vi "collectAI_tt.vi"() -> ()   [LabVIEW 2013]
uses:
  <vilib>/DAQmx/read.llb/DAQmx Read (Analog 2D I16 NChan NSamp).vi
  <vilib>/DAQmx/miscellaneous.llb/DAQmx Fill In Error Info.vi
panel:
  out "AIarray 2":bool[](array[boolean])
  out "AI?":bool
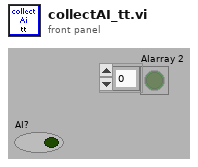
[diagram p1: front panel]
types:
  T1 = cluster{"StageS":i32, "StageL":i32, "data dir":path, "image OD":u16, "contour OD":u16, "point OD":u16, "AOlines":tag[], "AIlines":tag[], "CI lines":tag[], "DO lines":tag[], "AO names":string[], "CI names":string[], "AI names":string[], "DO names":string[]}
  T2 = typedef "LVRectTypeDef.ctl" = cluster{"Left":i16, "Top":i16, "Right":i16, "Bottom":i16}
  T3 = cluster{"Xpixels":i32, "Vxminref":dbl, "Vxmaxref":dbl, "P":dbl, "Ypixels":i32, "Vyminref":dbl, "Vymaxref":dbl, "srate":sgl, "sAOxy":i32, "timeout":dbl, "type":string, "date":string, "time":string, "Colormap":u16, "Drawing Mode":u16, "Scanning Mode":u16, "square pixels":bool, "square matrix":bool, "Xpixels Img":i32, "Vx-min Img":dbl, "VX-max Img":dbl, "Ypixels Img":i32, "Vy-min Img":dbl, "Vy-max Img ":dbl, "Angle Img":dbl, "autoshutter":bool, "finite":bool, "cont":bool, "wavdet":bool, "measpoints":i32, "avpp":i32, "bufferAO":i32, "bufferAI":i32, "starttick":u32, "waveform":path, "Vx-ref":dbl, "Vy-ref":dbl, "refreshrate":dbl, "refreshbuffer":i32, "tt_cycles":i32, "motorref":refnum<k7>, "mirrorswitch":refnum<k7>, "sample mode":i32, "maxbufferAI":i32, "sampletreshold":dbl, "srateAODO":sgl, "bin":sgl, "Pel":sgl, "Angle draw":dbl, "srate Img":sgl, "ROIimg_plotbounds":T2, "auto OD":bool, "ODfilt":u16, "reset AO_DO":bool, "aAI":i32[], "aCI":i32[], "aAO":i32[], "aDO":i32[]}
  T4 = cluster{" AI":refnum<k21>, "E_AI":errorcluster, "header":dbl[]}
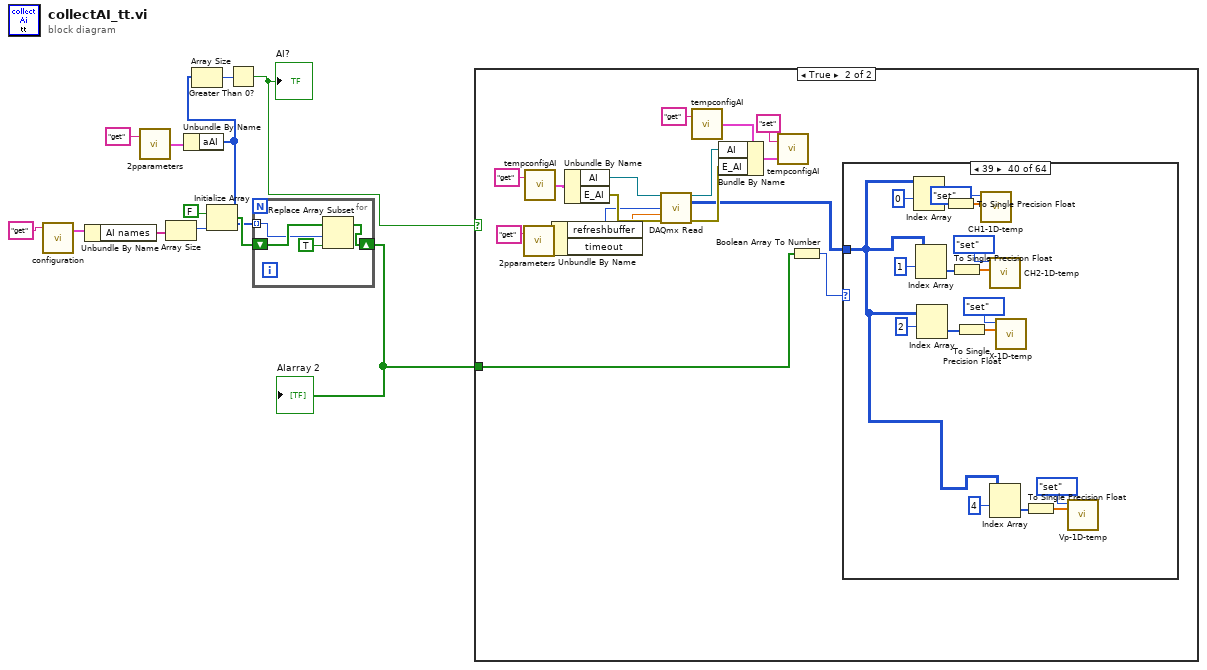
[diagram p0: block diagram]
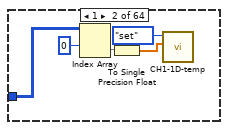
[diagram p4: hidden frame]
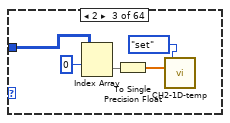
[diagram p5: hidden frame]
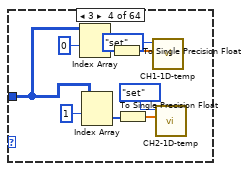
[diagram p6: hidden frame]
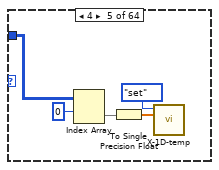
[diagram p7: hidden frame]
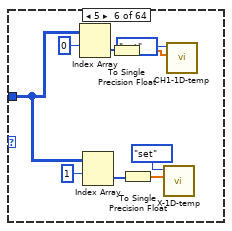
[diagram p8: hidden frame]
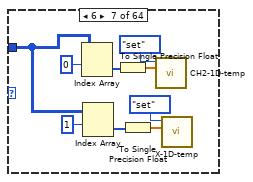
[diagram p9: hidden frame]
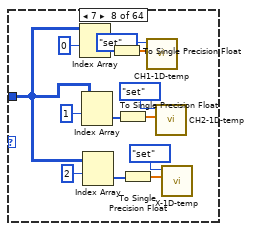
[diagram p10: hidden frame]
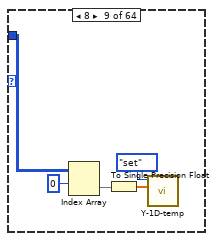
[diagram p11: hidden frame]
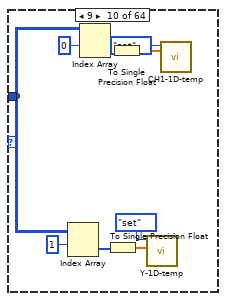
[diagram p12: hidden frame]
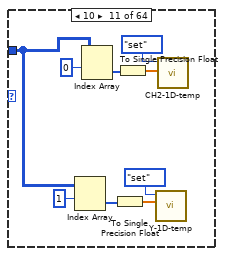
[diagram p13: hidden frame]
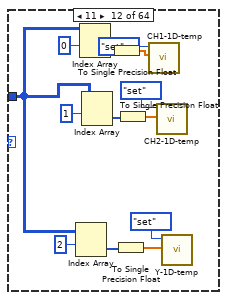
[diagram p14: hidden frame]
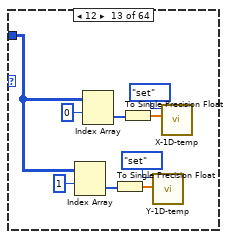
[diagram p15: hidden frame]
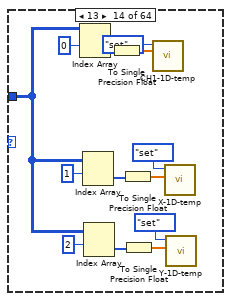
[diagram p16: hidden frame]
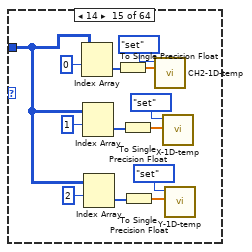
[diagram p17: hidden frame]
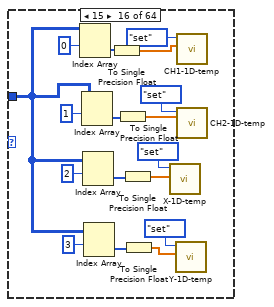
[diagram p18: hidden frame]
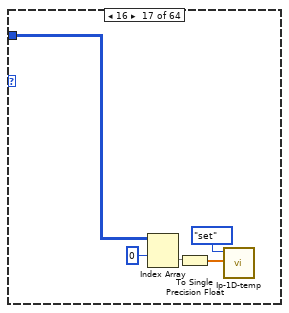
[diagram p19: hidden frame]
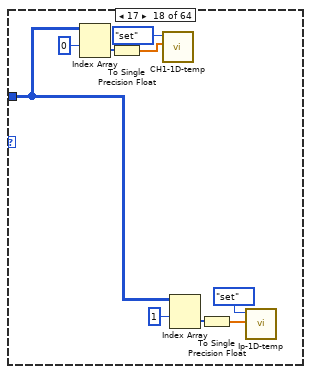
[diagram p20: hidden frame]
diagram:
  n1 = call "configuration.vi"("command"="get") -> ("config out"=w9:T1)  [unwired: 2 in, 1 out]
  n2 = Unbundle By Name(w9) -> ("AI names"=w8:string[])
  n3 = call "2pparameters.vi"("command"="get") -> ("params out"=w10:T3)  [unwired: 1 in]
  n4 = Array Size(array=w8) -> (size(s)=w7:i32)
  n5 = Unbundle By Name(w10) -> ("aAI"=w4:i32[])
  n6 = Array Size(array=w4) -> (size(s)=w3:i32)
  n7 = Initialize Array(FALSE, w7) -> (w5:bool[])
  n8 = Greater Than 0?(x=w3) -> (x > 0?=w2:bool)
  "AI?" <- w2
  n9 = for {
    tunnel: w4 -> [w15] mode=indexing
    shift-right: [w13] -> w1
    shift-left: w5 -> [w16]
    n10 = Replace Array Subset(array=w16, new element=TRUE ("new element/subarray"), index=w15) -> (w13:bool[])
  }
  "AIarray 2" <- w1
  n11 = case shown="True" w2 {
    tunnel: w1 -> [_ w18]
    frame False {
    }
    frame True {
      n12 = call "2pparameters.vi"("command"="get") -> ("params out"=w20:T3)  [unwired: 1 in]
      n13 = call "tempconfigAI.vi"("command"="get") -> ("Temp Config out"=w30:T4)  [unwired: 1 in]
      n14 = Unbundle By Name(w20) -> ("refreshbuffer"=w23:i32, "timeout"=w22:dbl)
      n15 = Unbundle By Name(w30) -> ("AI"=w29:refnum<k21>, "E_AI"=w28:errorcluster)
      n16 = call-poly <vilib>:"DAQmx Read.vi"("task/channels in"=w29, "number of samples per channel"=w23, "timeout"=w22, "error in"=w28) -> ("task out"=w24:refnum<k21>, "data"=w17:i16[][], "error out"=w33:errorcluster)  [unwired: 9 in]
      n17 = call "tempconfigAI.vi"("command"="get") -> ("Temp Config out"=w25:T4)  [unwired: 1 in]
      n18 = Bundle By Name(cluster=w25, "AI"=w24, "E_AI"=w33) -> (w32:T4)
      n19 = call "tempconfigAI.vi"("Temp Config in"=w32, "command"="set") -> ()  [unwired: 1 out]
      n20 = Boolean Array To Number(Boolean array=w18) -> (number=w19:u32)
      n21 = case shown="39" w19 {
        tunnel: w17 -> [_ w38 w43 w52 w57 w62 w71 w88 w93 w102 w111 w124 w129 w146 w159 w176 w177 w182 w191 w200 w213 w222 w235 w248 w265 w274 w287 w300 w317 w330 w347 w364 w385 w390 w399 w408 w421 w430 w443 w456 w473 w482 w495 w508 w525 w538 w555 w572 w593 w602 w615 w628 w645 w658 w675 w692 w713 w726 w743 w760 w781 w798 w819 w840]
        frame 0, Default {
        }
        frame 1 {
          n22 = Index Array(array=w38, index (row)=0) -> (element=w36:i16[])  [unwired: 1 in]
          n23 = To Single Precision Float(number=w36) -> (single precision float=w34:sgl[])
          n24 = call "CH1-1D-temp.vi"("array in"=w34, "command"=enum16{"get", "set", "clear", "append"}."set") -> ()  [unwired: 2 in, 2 out]
        }
        frame 2 {
          n25 = Index Array(array=w43, index (row)=0) -> (element=w41:i16[])  [unwired: 1 in]
          n26 = To Single Precision Float(number=w41) -> (single precision float=w40:sgl[])
          n27 = call "CH2-1D-temp.vi"("array in"=w40, "command"=enum16{"get", "set", "clear", "append"}."set") -> ()  [unwired: 2 in, 2 out]
        }
        frame 3 {
          n28 = Index Array(array=w52, index (row)=0) -> (element=w49:i16[])  [unwired: 1 in]
          n29 = Index Array(array=w52, index (row)=1) -> (element=w48:i16[])  [unwired: 1 in]
          n30 = To Single Precision Float(number=w49) -> (single precision float=w46:sgl[])
          n31 = To Single Precision Float(number=w48) -> (single precision float=w44:sgl[])
          n32 = call "CH1-1D-temp.vi"("array in"=w46, "command"=enum16{"get", "set", "clear", "append"}."set") -> ()  [unwired: 2 in, 2 out]
          n33 = call "CH2-1D-temp.vi"("array in"=w44, "command"=enum16{"get", "set", "clear", "append"}."set") -> ()  [unwired: 2 in, 2 out]
        }
        frame 4 {
          n34 = Index Array(array=w57, index (row)=0) -> (element=w55:i16[])  [unwired: 1 in]
          n35 = To Single Precision Float(number=w55) -> (single precision float=w53:sgl[])
          n36 = call "X-1D-temp.vi"("array in"=w53, "command"=enum16{"get", "set", "clear", "append"}."set") -> ()  [unwired: 2 in, 2 out]
        }
        frame 5 {
          n37 = Index Array(array=w62, index (row)=0) -> (element=w64:i16[])  [unwired: 1 in]
          n38 = Index Array(array=w62, index (row)=1) -> (element=w63:i16[])  [unwired: 1 in]
          n39 = To Single Precision Float(number=w64) -> (single precision float=w60:sgl[])
          n40 = To Single Precision Float(number=w63) -> (single precision float=w58:sgl[])
          n41 = call "X-1D-temp.vi"("array in"=w58, "command"=enum16{"get", "set", "clear", "append"}."set") -> ()  [unwired: 2 in, 2 out]
          n42 = call "CH1-1D-temp.vi"("array in"=w60, "command"=enum16{"get", "set", "clear", "append"}."set") -> ()  [unwired: 2 in, 2 out]
        }
        frame 6 {
          n43 = Index Array(array=w71, index (row)=0) -> (element=w73:i16[])  [unwired: 1 in]
          n44 = Index Array(array=w71, index (row)=1) -> (element=w72:i16[])  [unwired: 1 in]
          n45 = To Single Precision Float(number=w73) -> (single precision float=w69:sgl[])
          n46 = To Single Precision Float(number=w72) -> (single precision float=w67:sgl[])
          n47 = call "CH2-1D-temp.vi"("array in"=w69, "command"=enum16{"get", "set", "clear", "append"}."set") -> ()  [unwired: 2 in, 2 out]
          n48 = call "X-1D-temp.vi"("array in"=w67, "command"=enum16{"get", "set", "clear", "append"}."set") -> ()  [unwired: 2 in, 2 out]
        }
        frame 7 {
          n49 = Index Array(array=w88, index (row)=0) -> (element=w84:i16[])  [unwired: 1 in]
          n50 = Index Array(array=w88, index (row)=1) -> (element=w83:i16[])  [unwired: 1 in]
          n51 = Index Array(array=w88, index (row)=2) -> (element=w82:i16[])  [unwired: 1 in]
          n52 = To Single Precision Float(number=w84) -> (single precision float=w80:sgl[])
          n53 = To Single Precision Float(number=w83) -> (single precision float=w78:sgl[])
          n54 = To Single Precision Float(number=w82) -> (single precision float=w76:sgl[])
          n55 = call "CH1-1D-temp.vi"("array in"=w80, "command"=enum16{"get", "set", "clear", "append"}."set") -> ()  [unwired: 2 in, 2 out]
          n56 = call "CH2-1D-temp.vi"("array in"=w78, "command"=enum16{"get", "set", "clear", "append"}."set") -> ()  [unwired: 2 in, 2 out]
          n57 = call "X-1D-temp.vi"("array in"=w76, "command"=enum16{"get", "set", "clear", "append"}."set") -> ()  [unwired: 2 in, 2 out]
        }
        frame 8 {
          n58 = Index Array(array=w93, index (row)=0) -> (element=w92:i16[])  [unwired: 1 in]
          n59 = To Single Precision Float(number=w92) -> (single precision float=w89:sgl[])
          n60 = call "Y-1D-temp.vi"("array in"=w89, "command"=enum16{"get", "set", "clear", "append"}."set") -> ()  [unwired: 2 in, 2 out]
        }
        frame 9 {
          n61 = Index Array(array=w102, index (row)=1) -> (element=w99:i16[])  [unwired: 1 in]
          n62 = Index Array(array=w102, index (row)=0) -> (element=w100:i16[])  [unwired: 1 in]
          n63 = To Single Precision Float(number=w99) -> (single precision float=w94:sgl[])
          n64 = To Single Precision Float(number=w100) -> (single precision float=w96:sgl[])
          n65 = call "Y-1D-temp.vi"("array in"=w94, "command"=enum16{"get", "set", "clear", "append"}."set") -> ()  [unwired: 2 in, 2 out]
          n66 = call "CH1-1D-temp.vi"("array in"=w96, "command"=enum16{"get", "set", "clear", "append"}."set") -> ()  [unwired: 2 in, 2 out]
        }
        frame 10 {
          n67 = Index Array(array=w111, index (row)=1) -> (element=w108:i16[])  [unwired: 1 in]
          n68 = Index Array(array=w111, index (row)=0) -> (element=w109:i16[])  [unwired: 1 in]
          n69 = To Single Precision Float(number=w108) -> (single precision float=w103:sgl[])
          n70 = To Single Precision Float(number=w109) -> (single precision float=w106:sgl[])
          n71 = call "Y-1D-temp.vi"("array in"=w103, "command"=enum16{"get", "set", "clear", "append"}."set") -> ()  [unwired: 2 in, 2 out]
          n72 = call "CH2-1D-temp.vi"("array in"=w106, "command"=enum16{"get", "set", "clear", "append"}."set") -> ()  [unwired: 2 in, 2 out]
        }
        frame 11 {
          n73 = Index Array(array=w124, index (row)=2) -> (element=w119:i16[])  [unwired: 1 in]
          n74 = Index Array(array=w124, index (row)=0) -> (element=w121:i16[])  [unwired: 1 in]
          n75 = Index Array(array=w124, index (row)=1) -> (element=w120:i16[])  [unwired: 1 in]
          n76 = To Single Precision Float(number=w121) -> (single precision float=w116:sgl[])
          n77 = To Single Precision Float(number=w119) -> (single precision float=w113:sgl[])
          n78 = To Single Precision Float(number=w120) -> (single precision float=w114:sgl[])
          n79 = call "CH1-1D-temp.vi"("array in"=w116, "command"=enum16{"get", "set", "clear", "append"}."set") -> ()  [unwired: 2 in, 2 out]
          n80 = call "CH2-1D-temp.vi"("array in"=w114, "command"=enum16{"get", "set", "clear", "append"}."set") -> ()  [unwired: 2 in, 2 out]
          n81 = call "Y-1D-temp.vi"("array in"=w113, "command"=enum16{"get", "set", "clear", "append"}."set") -> ()  [unwired: 2 in, 2 out]
        }
        frame 12 {
          n82 = Index Array(array=w129, index (row)=1) -> (element=w131:i16[])  [unwired: 1 in]
          n83 = Index Array(array=w129, index (row)=0) -> (element=w132:i16[])  [unwired: 1 in]
          n84 = To Single Precision Float(number=w131) -> (single precision float=w125:sgl[])
          n85 = To Single Precision Float(number=w132) -> (single precision float=w127:sgl[])
          n86 = call "Y-1D-temp.vi"("array in"=w125, "command"=enum16{"get", "set", "clear", "append"}."set") -> ()  [unwired: 2 in, 2 out]
          n87 = call "X-1D-temp.vi"("array in"=w127, "command"=enum16{"get", "set", "clear", "append"}."set") -> ()  [unwired: 2 in, 2 out]
        }
        frame 13 {
          n88 = Index Array(array=w146, index (row)=0) -> (element=w143:i16[])  [unwired: 1 in]
          n89 = Index Array(array=w146, index (row)=1) -> (element=w142:i16[])  [unwired: 1 in]
          n90 = Index Array(array=w146, index (row)=2) -> (element=w141:i16[])  [unwired: 1 in]
          n91 = To Single Precision Float(number=w143) -> (single precision float=w138:sgl[])
          n92 = To Single Precision Float(number=w142) -> (single precision float=w136:sgl[])
          n93 = To Single Precision Float(number=w141) -> (single precision float=w134:sgl[])
          n94 = call "CH1-1D-temp.vi"("array in"=w138, "command"=enum16{"get", "set", "clear", "append"}."set") -> ()  [unwired: 2 in, 2 out]
          n95 = call "X-1D-temp.vi"("array in"=w136, "command"=enum16{"get", "set", "clear", "append"}."set") -> ()  [unwired: 2 in, 2 out]
          n96 = call "Y-1D-temp.vi"("array in"=w134, "command"=enum16{"get", "set", "clear", "append"}."set") -> ()  [unwired: 2 in, 2 out]
        }
        frame 14 {
          n97 = Index Array(array=w159, index (row)=0) -> (element=w156:i16[])  [unwired: 1 in]
          n98 = Index Array(array=w159, index (row)=1) -> (element=w155:i16[])  [unwired: 1 in]
          n99 = Index Array(array=w159, index (row)=2) -> (element=w154:i16[])  [unwired: 1 in]
          n100 = To Single Precision Float(number=w156) -> (single precision float=w151:sgl[])
          n101 = To Single Precision Float(number=w155) -> (single precision float=w149:sgl[])
          n102 = To Single Precision Float(number=w154) -> (single precision float=w147:sgl[])
          n103 = call "CH2-1D-temp.vi"("array in"=w151, "command"=enum16{"get", "set", "clear", "append"}."set") -> ()  [unwired: 2 in, 2 out]
          n104 = call "X-1D-temp.vi"("array in"=w149, "command"=enum16{"get", "set", "clear", "append"}."set") -> ()  [unwired: 2 in, 2 out]
          n105 = call "Y-1D-temp.vi"("array in"=w147, "command"=enum16{"get", "set", "clear", "append"}."set") -> ()  [unwired: 2 in, 2 out]
        }
        frame 15 {
          n106 = Index Array(array=w176, index (row)=0) -> (element=w172:i16[])  [unwired: 1 in]
          n107 = Index Array(array=w176, index (row)=1) -> (element=w171:i16[])  [unwired: 1 in]
          n108 = Index Array(array=w176, index (row)=2) -> (element=w170:i16[])  [unwired: 1 in]
          n109 = Index Array(array=w176, index (row)=3) -> (element=w169:i16[])  [unwired: 1 in]
          n110 = To Single Precision Float(number=w172) -> (single precision float=w166:sgl[])
          n111 = To Single Precision Float(number=w171) -> (single precision float=w164:sgl[])
          n112 = To Single Precision Float(number=w170) -> (single precision float=w162:sgl[])
          n113 = To Single Precision Float(number=w169) -> (single precision float=w160:sgl[])
          n114 = call "X-1D-temp.vi"("array in"=w162, "command"=enum16{"get", "set", "clear", "append"}."set") -> ()  [unwired: 2 in, 2 out]
          n115 = call "Y-1D-temp.vi"("array in"=w160, "command"=enum16{"get", "set", "clear", "append"}."set") -> ()  [unwired: 2 in, 2 out]
          n116 = call "CH1-1D-temp.vi"("array in"=w166, "command"=enum16{"get", "set", "clear", "append"}."set") -> ()  [unwired: 2 in, 2 out]
          n117 = call "CH2-1D-temp.vi"("array in"=w164, "command"=enum16{"get", "set", "clear", "append"}."set") -> ()  [unwired: 2 in, 2 out]
        }
        frame 16 {
          n118 = Index Array(array=w177, index (row)=0) -> (element=w180:i16[])  [unwired: 1 in]
          n119 = To Single Precision Float(number=w180) -> (single precision float=w178:sgl[])
          n120 = call "Ip-1D-temp.vi"("array in"=w178, "command"=enum16{"get", "set", "clear", "append"}."set") -> ()  [unwired: 2 in, 2 out]
        }
        frame 17 {
          n121 = Index Array(array=w182, index (row)=0) -> (element=w189:i16[])  [unwired: 1 in]
          n122 = To Single Precision Float(number=w189) -> (single precision float=w187:sgl[])
          n123 = call "CH1-1D-temp.vi"("array in"=w187, "command"=enum16{"get", "set", "clear", "append"}."set") -> ()  [unwired: 2 in, 2 out]
          n124 = Index Array(array=w182, index (row)=1) -> (element=w185:i16[])  [unwired: 1 in]
          n125 = To Single Precision Float(number=w185) -> (single precision float=w183:sgl[])
          n126 = call "Ip-1D-temp.vi"("array in"=w183, "command"=enum16{"get", "set", "clear", "append"}."set") -> ()  [unwired: 2 in, 2 out]
        }
        frame 18 {
          n127 = Index Array(array=w191, index (row)=0) -> (element=w198:i16[])  [unwired: 1 in]
          n128 = To Single Precision Float(number=w198) -> (single precision float=w197:sgl[])
          n129 = Index Array(array=w191, index (row)=1) -> (element=w194:i16[])  [unwired: 1 in]
          n130 = call "CH2-1D-temp.vi"("array in"=w197, "command"=enum16{"get", "set", "clear", "append"}."set") -> ()  [unwired: 2 in, 2 out]
          n131 = To Single Precision Float(number=w194) -> (single precision float=w192:sgl[])
          n132 = call "Ip-1D-temp.vi"("array in"=w192, "command"=enum16{"get", "set", "clear", "append"}."set") -> ()  [unwired: 2 in, 2 out]
        }
        frame 19 {
          n133 = Index Array(array=w200, index (row)=0) -> (element=w210:i16[])  [unwired: 1 in]
          n134 = Index Array(array=w200, index (row)=1) -> (element=w209:i16[])  [unwired: 1 in]
          n135 = To Single Precision Float(number=w210) -> (single precision float=w207:sgl[])
          n136 = To Single Precision Float(number=w209) -> (single precision float=w205:sgl[])
          n137 = call "CH1-1D-temp.vi"("array in"=w207, "command"=enum16{"get", "set", "clear", "append"}."set") -> ()  [unwired: 2 in, 2 out]
          n138 = call "CH2-1D-temp.vi"("array in"=w205, "command"=enum16{"get", "set", "clear", "append"}."set") -> ()  [unwired: 2 in, 2 out]
          n139 = Index Array(array=w200, index (row)=2) -> (element=w203:i16[])  [unwired: 1 in]
          n140 = To Single Precision Float(number=w203) -> (single precision float=w201:sgl[])
          n141 = call "Ip-1D-temp.vi"("array in"=w201, "command"=enum16{"get", "set", "clear", "append"}."set") -> ()  [unwired: 2 in, 2 out]
        }
        frame 20 {
          n142 = Index Array(array=w213, index (row)=0) -> (element=w220:i16[])  [unwired: 1 in]
          n143 = To Single Precision Float(number=w220) -> (single precision float=w218:sgl[])
          n144 = Index Array(array=w213, index (row)=1) -> (element=w216:i16[])  [unwired: 1 in]
          n145 = call "X-1D-temp.vi"("array in"=w218, "command"=enum16{"get", "set", "clear", "append"}."set") -> ()  [unwired: 2 in, 2 out]
          n146 = To Single Precision Float(number=w216) -> (single precision float=w214:sgl[])
          n147 = call "Ip-1D-temp.vi"("array in"=w214, "command"=enum16{"get", "set", "clear", "append"}."set") -> ()  [unwired: 2 in, 2 out]
        }
        frame 21 {
          n148 = Index Array(array=w222, index (row)=0) -> (element=w232:i16[])  [unwired: 1 in]
          n149 = Index Array(array=w222, index (row)=1) -> (element=w231:i16[])  [unwired: 1 in]
          n150 = To Single Precision Float(number=w232) -> (single precision float=w229:sgl[])
          n151 = To Single Precision Float(number=w231) -> (single precision float=w227:sgl[])
          n152 = Index Array(array=w222, index (row)=2) -> (element=w225:i16[])  [unwired: 1 in]
          n153 = call "X-1D-temp.vi"("array in"=w227, "command"=enum16{"get", "set", "clear", "append"}."set") -> ()  [unwired: 2 in, 2 out]
          n154 = call "CH1-1D-temp.vi"("array in"=w229, "command"=enum16{"get", "set", "clear", "append"}."set") -> ()  [unwired: 2 in, 2 out]
          n155 = To Single Precision Float(number=w225) -> (single precision float=w223:sgl[])
          n156 = call "Ip-1D-temp.vi"("array in"=w223, "command"=enum16{"get", "set", "clear", "append"}."set") -> ()  [unwired: 2 in, 2 out]
        }
        frame 22 {
          n157 = Index Array(array=w235, index (row)=0) -> (element=w245:i16[])  [unwired: 1 in]
          n158 = Index Array(array=w235, index (row)=1) -> (element=w244:i16[])  [unwired: 1 in]
          n159 = To Single Precision Float(number=w245) -> (single precision float=w242:sgl[])
          n160 = To Single Precision Float(number=w244) -> (single precision float=w240:sgl[])
          n161 = Index Array(array=w235, index (row)=2) -> (element=w238:i16[])  [unwired: 1 in]
          n162 = call "CH2-1D-temp.vi"("array in"=w242, "command"=enum16{"get", "set", "clear", "append"}."set") -> ()  [unwired: 2 in, 2 out]
          n163 = To Single Precision Float(number=w238) -> (single precision float=w236:sgl[])
          n164 = call "X-1D-temp.vi"("array in"=w240, "command"=enum16{"get", "set", "clear", "append"}."set") -> ()  [unwired: 2 in, 2 out]
          n165 = call "Ip-1D-temp.vi"("array in"=w236, "command"=enum16{"get", "set", "clear", "append"}."set") -> ()  [unwired: 2 in, 2 out]
        }
        frame 23 {
          n166 = Index Array(array=w248, index (row)=0) -> (element=w261:i16[])  [unwired: 1 in]
          n167 = Index Array(array=w248, index (row)=1) -> (element=w260:i16[])  [unwired: 1 in]
          n168 = Index Array(array=w248, index (row)=2) -> (element=w259:i16[])  [unwired: 1 in]
          n169 = To Single Precision Float(number=w261) -> (single precision float=w257:sgl[])
          n170 = To Single Precision Float(number=w260) -> (single precision float=w255:sgl[])
          n171 = To Single Precision Float(number=w259) -> (single precision float=w253:sgl[])
          n172 = call "CH1-1D-temp.vi"("array in"=w257, "command"=enum16{"get", "set", "clear", "append"}."set") -> ()  [unwired: 2 in, 2 out]
          n173 = Index Array(array=w248, index (row)=3) -> (element=w251:i16[])  [unwired: 1 in]
          n174 = call "CH2-1D-temp.vi"("array in"=w255, "command"=enum16{"get", "set", "clear", "append"}."set") -> ()  [unwired: 2 in, 2 out]
          n175 = call "X-1D-temp.vi"("array in"=w253, "command"=enum16{"get", "set", "clear", "append"}."set") -> ()  [unwired: 2 in, 2 out]
          n176 = To Single Precision Float(number=w251) -> (single precision float=w249:sgl[])
          n177 = call "Ip-1D-temp.vi"("array in"=w249, "command"=enum16{"get", "set", "clear", "append"}."set") -> ()  [unwired: 2 in, 2 out]
        }
        frame 24 {
          n178 = Index Array(array=w265, index (row)=0) -> (element=w273:i16[])  [unwired: 1 in]
          n179 = To Single Precision Float(number=w273) -> (single precision float=w270:sgl[])
          n180 = call "Y-1D-temp.vi"("array in"=w270, "command"=enum16{"get", "set", "clear", "append"}."set") -> ()  [unwired: 2 in, 2 out]
          n181 = Index Array(array=w265, index (row)=1) -> (element=w268:i16[])  [unwired: 1 in]
          n182 = To Single Precision Float(number=w268) -> (single precision float=w266:sgl[])
          n183 = call "Ip-1D-temp.vi"("array in"=w266, "command"=enum16{"get", "set", "clear", "append"}."set") -> ()  [unwired: 2 in, 2 out]
        }
        frame 25 {
          n184 = Index Array(array=w274, index (row)=1) -> (element=w284:i16[])  [unwired: 1 in]
          n185 = Index Array(array=w274, index (row)=0) -> (element=w285:i16[])  [unwired: 1 in]
          n186 = To Single Precision Float(number=w284) -> (single precision float=w279:sgl[])
          n187 = To Single Precision Float(number=w285) -> (single precision float=w281:sgl[])
          n188 = call "Y-1D-temp.vi"("array in"=w279, "command"=enum16{"get", "set", "clear", "append"}."set") -> ()  [unwired: 2 in, 2 out]
          n189 = call "CH1-1D-temp.vi"("array in"=w281, "command"=enum16{"get", "set", "clear", "append"}."set") -> ()  [unwired: 2 in, 2 out]
          n190 = Index Array(array=w274, index (row)=2) -> (element=w277:i16[])  [unwired: 1 in]
          n191 = To Single Precision Float(number=w277) -> (single precision float=w275:sgl[])
          n192 = call "Ip-1D-temp.vi"("array in"=w275, "command"=enum16{"get", "set", "clear", "append"}."set") -> ()  [unwired: 2 in, 2 out]
        }
        frame 26 {
          n193 = Index Array(array=w287, index (row)=1) -> (element=w297:i16[])  [unwired: 1 in]
          n194 = Index Array(array=w287, index (row)=0) -> (element=w298:i16[])  [unwired: 1 in]
          n195 = To Single Precision Float(number=w297) -> (single precision float=w292:sgl[])
          n196 = To Single Precision Float(number=w298) -> (single precision float=w295:sgl[])
          n197 = call "Y-1D-temp.vi"("array in"=w292, "command"=enum16{"get", "set", "clear", "append"}."set") -> ()  [unwired: 2 in, 2 out]
          n198 = call "CH2-1D-temp.vi"("array in"=w295, "command"=enum16{"get", "set", "clear", "append"}."set") -> ()  [unwired: 2 in, 2 out]
          n199 = Index Array(array=w287, index (row)=2) -> (element=w290:i16[])  [unwired: 1 in]
          n200 = To Single Precision Float(number=w290) -> (single precision float=w288:sgl[])
          n201 = call "Ip-1D-temp.vi"("array in"=w288, "command"=enum16{"get", "set", "clear", "append"}."set") -> ()  [unwired: 2 in, 2 out]
        }
        frame 27 {
          n202 = Index Array(array=w300, index (row)=2) -> (element=w312:i16[])  [unwired: 1 in]
          n203 = Index Array(array=w300, index (row)=0) -> (element=w314:i16[])  [unwired: 1 in]
          n204 = Index Array(array=w300, index (row)=1) -> (element=w313:i16[])  [unwired: 1 in]
          n205 = To Single Precision Float(number=w314) -> (single precision float=w309:sgl[])
          n206 = To Single Precision Float(number=w312) -> (single precision float=w306:sgl[])
          n207 = To Single Precision Float(number=w313) -> (single precision float=w307:sgl[])
          n208 = call "CH1-1D-temp.vi"("array in"=w309, "command"=enum16{"get", "set", "clear", "append"}."set") -> ()  [unwired: 2 in, 2 out]
          n209 = call "CH2-1D-temp.vi"("array in"=w307, "command"=enum16{"get", "set", "clear", "append"}."set") -> ()  [unwired: 2 in, 2 out]
          n210 = Index Array(array=w300, index (row)=3) -> (element=w303:i16[])  [unwired: 1 in]
          n211 = call "Y-1D-temp.vi"("array in"=w306, "command"=enum16{"get", "set", "clear", "append"}."set") -> ()  [unwired: 2 in, 2 out]
          n212 = To Single Precision Float(number=w303) -> (single precision float=w301:sgl[])
          n213 = call "Ip-1D-temp.vi"("array in"=w301, "command"=enum16{"get", "set", "clear", "append"}."set") -> ()  [unwired: 2 in, 2 out]
        }
        frame 28 {
          n214 = Index Array(array=w317, index (row)=1) -> (element=w327:i16[])  [unwired: 1 in]
          n215 = Index Array(array=w317, index (row)=0) -> (element=w328:i16[])  [unwired: 1 in]
          n216 = To Single Precision Float(number=w327) -> (single precision float=w322:sgl[])
          n217 = To Single Precision Float(number=w328) -> (single precision float=w324:sgl[])
          n218 = call "Y-1D-temp.vi"("array in"=w322, "command"=enum16{"get", "set", "clear", "append"}."set") -> ()  [unwired: 2 in, 2 out]
          n219 = Index Array(array=w317, index (row)=2) -> (element=w320:i16[])  [unwired: 1 in]
          n220 = call "X-1D-temp.vi"("array in"=w324, "command"=enum16{"get", "set", "clear", "append"}."set") -> ()  [unwired: 2 in, 2 out]
          n221 = To Single Precision Float(number=w320) -> (single precision float=w318:sgl[])
          n222 = call "Ip-1D-temp.vi"("array in"=w318, "command"=enum16{"get", "set", "clear", "append"}."set") -> ()  [unwired: 2 in, 2 out]
        }
        frame 29 {
          n223 = Index Array(array=w330, index (row)=0) -> (element=w344:i16[])  [unwired: 1 in]
          n224 = Index Array(array=w330, index (row)=1) -> (element=w343:i16[])  [unwired: 1 in]
          n225 = Index Array(array=w330, index (row)=2) -> (element=w342:i16[])  [unwired: 1 in]
          n226 = To Single Precision Float(number=w344) -> (single precision float=w339:sgl[])
          n227 = To Single Precision Float(number=w343) -> (single precision float=w337:sgl[])
          n228 = To Single Precision Float(number=w342) -> (single precision float=w335:sgl[])
          n229 = Index Array(array=w330, index (row)=3) -> (element=w333:i16[])  [unwired: 1 in]
          n230 = call "CH1-1D-temp.vi"("array in"=w339, "command"=enum16{"get", "set", "clear", "append"}."set") -> ()  [unwired: 2 in, 2 out]
          n231 = call "X-1D-temp.vi"("array in"=w337, "command"=enum16{"get", "set", "clear", "append"}."set") -> ()  [unwired: 2 in, 2 out]
          n232 = call "Y-1D-temp.vi"("array in"=w335, "command"=enum16{"get", "set", "clear", "append"}."set") -> ()  [unwired: 2 in, 2 out]
          n233 = To Single Precision Float(number=w333) -> (single precision float=w331:sgl[])
          n234 = call "Ip-1D-temp.vi"("array in"=w331, "command"=enum16{"get", "set", "clear", "append"}."set") -> ()  [unwired: 2 in, 2 out]
        }
        frame 30 {
          n235 = Index Array(array=w347, index (row)=3) -> (element=w350:i16[])  [unwired: 1 in]
          n236 = Index Array(array=w347, index (row)=0) -> (element=w361:i16[])  [unwired: 1 in]
          n237 = Index Array(array=w347, index (row)=1) -> (element=w360:i16[])  [unwired: 1 in]
          n238 = Index Array(array=w347, index (row)=2) -> (element=w359:i16[])  [unwired: 1 in]
          n239 = To Single Precision Float(number=w350) -> (single precision float=w348:sgl[])
          n240 = To Single Precision Float(number=w361) -> (single precision float=w356:sgl[])
          n241 = To Single Precision Float(number=w360) -> (single precision float=w354:sgl[])
          n242 = To Single Precision Float(number=w359) -> (single precision float=w352:sgl[])
          n243 = call "CH2-1D-temp.vi"("array in"=w356, "command"=enum16{"get", "set", "clear", "append"}."set") -> ()  [unwired: 2 in, 2 out]
          n244 = call "Ip-1D-temp.vi"("array in"=w348, "command"=enum16{"get", "set", "clear", "append"}."set") -> ()  [unwired: 2 in, 2 out]
          n245 = call "X-1D-temp.vi"("array in"=w354, "command"=enum16{"get", "set", "clear", "append"}."set") -> ()  [unwired: 2 in, 2 out]
          n246 = call "Y-1D-temp.vi"("array in"=w352, "command"=enum16{"get", "set", "clear", "append"}."set") -> ()  [unwired: 2 in, 2 out]
        }
        frame 31 {
          n247 = Index Array(array=w364, index (row)=0) -> (element=w381:i16[])  [unwired: 1 in]
          n248 = Index Array(array=w364, index (row)=1) -> (element=w380:i16[])  [unwired: 1 in]
          n249 = Index Array(array=w364, index (row)=2) -> (element=w379:i16[])  [unwired: 1 in]
          n250 = Index Array(array=w364, index (row)=3) -> (element=w378:i16[])  [unwired: 1 in]
          n251 = Index Array(array=w364, index (row)=4) -> (element=w367:i16[])  [unwired: 1 in]
          n252 = To Single Precision Float(number=w381) -> (single precision float=w375:sgl[])
          n253 = To Single Precision Float(number=w380) -> (single precision float=w373:sgl[])
          n254 = To Single Precision Float(number=w367) -> (single precision float=w365:sgl[])
          n255 = To Single Precision Float(number=w379) -> (single precision float=w371:sgl[])
          n256 = To Single Precision Float(number=w378) -> (single precision float=w369:sgl[])
          n257 = call "Ip-1D-temp.vi"("array in"=w365, "command"=enum16{"get", "set", "clear", "append"}."set") -> ()  [unwired: 2 in, 2 out]
          n258 = call "X-1D-temp.vi"("array in"=w371, "command"=enum16{"get", "set", "clear", "append"}."set") -> ()  [unwired: 2 in, 2 out]
          n259 = call "Y-1D-temp.vi"("array in"=w369, "command"=enum16{"get", "set", "clear", "append"}."set") -> ()  [unwired: 2 in, 2 out]
          n260 = call "CH1-1D-temp.vi"("array in"=w375, "command"=enum16{"get", "set", "clear", "append"}."set") -> ()  [unwired: 2 in, 2 out]
          n261 = call "CH2-1D-temp.vi"("array in"=w373, "command"=enum16{"get", "set", "clear", "append"}."set") -> ()  [unwired: 2 in, 2 out]
        }
        frame 32 {
          n262 = Index Array(array=w385, index (row)=1) -> (element=w388:i16[])  [unwired: 1 in]
          n263 = To Single Precision Float(number=w388) -> (single precision float=w386:sgl[])
          n264 = call "Vp-1D-temp.vi"("array in"=w386, "command"=enum16{"get", "set", "clear", "append"}."set") -> ()  [unwired: 2 in, 2 out]
        }
        frame 33 {
          n265 = Index Array(array=w390, index (row)=0) -> (element=w397:i16[])  [unwired: 1 in]
          n266 = To Single Precision Float(number=w397) -> (single precision float=w395:sgl[])
          n267 = call "CH1-1D-temp.vi"("array in"=w395, "command"=enum16{"get", "set", "clear", "append"}."set") -> ()  [unwired: 2 in, 2 out]
          n268 = Index Array(array=w390, index (row)=2) -> (element=w393:i16[])  [unwired: 1 in]
          n269 = To Single Precision Float(number=w393) -> (single precision float=w391:sgl[])
          n270 = call "Vp-1D-temp.vi"("array in"=w391, "command"=enum16{"get", "set", "clear", "append"}."set") -> ()  [unwired: 2 in, 2 out]
        }
        frame 34 {
          n271 = Index Array(array=w399, index (row)=0) -> (element=w406:i16[])  [unwired: 1 in]
          n272 = To Single Precision Float(number=w406) -> (single precision float=w405:sgl[])
          n273 = Index Array(array=w399, index (row)=2) -> (element=w402:i16[])  [unwired: 1 in]
          n274 = call "CH2-1D-temp.vi"("array in"=w405, "command"=enum16{"get", "set", "clear", "append"}."set") -> ()  [unwired: 2 in, 2 out]
          n275 = To Single Precision Float(number=w402) -> (single precision float=w400:sgl[])
          n276 = call "Vp-1D-temp.vi"("array in"=w400, "command"=enum16{"get", "set", "clear", "append"}."set") -> ()  [unwired: 2 in, 2 out]
        }
        frame 35 {
          n277 = Index Array(array=w408, index (row)=0) -> (element=w418:i16[])  [unwired: 1 in]
          n278 = Index Array(array=w408, index (row)=1) -> (element=w417:i16[])  [unwired: 1 in]
          n279 = To Single Precision Float(number=w418) -> (single precision float=w415:sgl[])
          n280 = To Single Precision Float(number=w417) -> (single precision float=w413:sgl[])
          n281 = call "CH1-1D-temp.vi"("array in"=w415, "command"=enum16{"get", "set", "clear", "append"}."set") -> ()  [unwired: 2 in, 2 out]
          n282 = call "CH2-1D-temp.vi"("array in"=w413, "command"=enum16{"get", "set", "clear", "append"}."set") -> ()  [unwired: 2 in, 2 out]
          n283 = Index Array(array=w408, index (row)=3) -> (element=w411:i16[])  [unwired: 1 in]
          n284 = To Single Precision Float(number=w411) -> (single precision float=w409:sgl[])
          n285 = call "Vp-1D-temp.vi"("array in"=w409, "command"=enum16{"get", "set", "clear", "append"}."set") -> ()  [unwired: 2 in, 2 out]
        }
        frame 36 {
          n286 = Index Array(array=w421, index (row)=0) -> (element=w428:i16[])  [unwired: 1 in]
          n287 = To Single Precision Float(number=w428) -> (single precision float=w426:sgl[])
          n288 = Index Array(array=w421, index (row)=2) -> (element=w424:i16[])  [unwired: 1 in]
          n289 = call "X-1D-temp.vi"("array in"=w426, "command"=enum16{"get", "set", "clear", "append"}."set") -> ()  [unwired: 2 in, 2 out]
          n290 = To Single Precision Float(number=w424) -> (single precision float=w422:sgl[])
          n291 = call "Vp-1D-temp.vi"("array in"=w422, "command"=enum16{"get", "set", "clear", "append"}."set") -> ()  [unwired: 2 in, 2 out]
        }
        frame 37 {
          n292 = Index Array(array=w430, index (row)=0) -> (element=w440:i16[])  [unwired: 1 in]
          n293 = Index Array(array=w430, index (row)=1) -> (element=w439:i16[])  [unwired: 1 in]
          n294 = To Single Precision Float(number=w440) -> (single precision float=w437:sgl[])
          n295 = To Single Precision Float(number=w439) -> (single precision float=w435:sgl[])
          n296 = Index Array(array=w430, index (row)=3) -> (element=w433:i16[])  [unwired: 1 in]
          n297 = call "X-1D-temp.vi"("array in"=w435, "command"=enum16{"get", "set", "clear", "append"}."set") -> ()  [unwired: 2 in, 2 out]
          n298 = call "CH1-1D-temp.vi"("array in"=w437, "command"=enum16{"get", "set", "clear", "append"}."set") -> ()  [unwired: 2 in, 2 out]
          n299 = To Single Precision Float(number=w433) -> (single precision float=w431:sgl[])
          n300 = call "Vp-1D-temp.vi"("array in"=w431, "command"=enum16{"get", "set", "clear", "append"}."set") -> ()  [unwired: 2 in, 2 out]
        }
        frame 38 {
          n301 = Index Array(array=w443, index (row)=0) -> (element=w453:i16[])  [unwired: 1 in]
          n302 = Index Array(array=w443, index (row)=1) -> (element=w452:i16[])  [unwired: 1 in]
          n303 = To Single Precision Float(number=w453) -> (single precision float=w450:sgl[])
          n304 = To Single Precision Float(number=w452) -> (single precision float=w448:sgl[])
          n305 = Index Array(array=w443, index (row)=3) -> (element=w446:i16[])  [unwired: 1 in]
          n306 = call "CH2-1D-temp.vi"("array in"=w450, "command"=enum16{"get", "set", "clear", "append"}."set") -> ()  [unwired: 2 in, 2 out]
          n307 = call "X-1D-temp.vi"("array in"=w448, "command"=enum16{"get", "set", "clear", "append"}."set") -> ()  [unwired: 2 in, 2 out]
          n308 = To Single Precision Float(number=w446) -> (single precision float=w444:sgl[])
          n309 = call "Vp-1D-temp.vi"("array in"=w444, "command"=enum16{"get", "set", "clear", "append"}."set") -> ()  [unwired: 2 in, 2 out]
        }
        frame 39 {
          n310 = Index Array(array=w456, index (row)=0) -> (element=w469:i16[])  [unwired: 1 in]
          n311 = Index Array(array=w456, index (row)=1) -> (element=w468:i16[])  [unwired: 1 in]
          n312 = Index Array(array=w456, index (row)=2) -> (element=w467:i16[])  [unwired: 1 in]
          n313 = To Single Precision Float(number=w469) -> (single precision float=w465:sgl[])
          n314 = To Single Precision Float(number=w468) -> (single precision float=w463:sgl[])
          n315 = To Single Precision Float(number=w467) -> (single precision float=w461:sgl[])
          n316 = call "CH1-1D-temp.vi"("array in"=w465, "command"=enum16{"get", "set", "clear", "append"}."set") -> ()  [unwired: 2 in, 2 out]
          n317 = call "CH2-1D-temp.vi"("array in"=w463, "command"=enum16{"get", "set", "clear", "append"}."set") -> ()  [unwired: 2 in, 2 out]
          n318 = Index Array(array=w456, index (row)=4) -> (element=w459:i16[])  [unwired: 1 in]
          n319 = call "X-1D-temp.vi"("array in"=w461, "command"=enum16{"get", "set", "clear", "append"}."set") -> ()  [unwired: 2 in, 2 out]
          n320 = To Single Precision Float(number=w459) -> (single precision float=w457:sgl[])
          n321 = call "Vp-1D-temp.vi"("array in"=w457, "command"=enum16{"get", "set", "clear", "append"}."set") -> ()  [unwired: 2 in, 2 out]
        }
        frame 40 {
          n322 = Index Array(array=w473, index (row)=0) -> (element=w481:i16[])  [unwired: 1 in]
          n323 = To Single Precision Float(number=w481) -> (single precision float=w478:sgl[])
          n324 = call "Y-1D-temp.vi"("array in"=w478, "command"=enum16{"get", "set", "clear", "append"}."set") -> ()  [unwired: 2 in, 2 out]
          n325 = Index Array(array=w473, index (row)=2) -> (element=w476:i16[])  [unwired: 1 in]
          n326 = To Single Precision Float(number=w476) -> (single precision float=w474:sgl[])
          n327 = call "Vp-1D-temp.vi"("array in"=w474, "command"=enum16{"get", "set", "clear", "append"}."set") -> ()  [unwired: 2 in, 2 out]
        }
        frame 41 {
          n328 = Index Array(array=w482, index (row)=1) -> (element=w492:i16[])  [unwired: 1 in]
          n329 = Index Array(array=w482, index (row)=0) -> (element=w493:i16[])  [unwired: 1 in]
          n330 = To Single Precision Float(number=w492) -> (single precision float=w487:sgl[])
          n331 = To Single Precision Float(number=w493) -> (single precision float=w489:sgl[])
          n332 = call "Y-1D-temp.vi"("array in"=w487, "command"=enum16{"get", "set", "clear", "append"}."set") -> ()  [unwired: 2 in, 2 out]
          n333 = call "CH1-1D-temp.vi"("array in"=w489, "command"=enum16{"get", "set", "clear", "append"}."set") -> ()  [unwired: 2 in, 2 out]
          n334 = Index Array(array=w482, index (row)=3) -> (element=w485:i16[])  [unwired: 1 in]
          n335 = To Single Precision Float(number=w485) -> (single precision float=w483:sgl[])
          n336 = call "Vp-1D-temp.vi"("array in"=w483, "command"=enum16{"get", "set", "clear", "append"}."set") -> ()  [unwired: 2 in, 2 out]
        }
        frame 42 {
          n337 = Index Array(array=w495, index (row)=1) -> (element=w505:i16[])  [unwired: 1 in]
          n338 = Index Array(array=w495, index (row)=0) -> (element=w506:i16[])  [unwired: 1 in]
          n339 = To Single Precision Float(number=w505) -> (single precision float=w500:sgl[])
          n340 = To Single Precision Float(number=w506) -> (single precision float=w503:sgl[])
          n341 = call "Y-1D-temp.vi"("array in"=w500, "command"=enum16{"get", "set", "clear", "append"}."set") -> ()  [unwired: 2 in, 2 out]
          n342 = call "CH2-1D-temp.vi"("array in"=w503, "command"=enum16{"get", "set", "clear", "append"}."set") -> ()  [unwired: 2 in, 2 out]
          n343 = Index Array(array=w495, index (row)=3) -> (element=w498:i16[])  [unwired: 1 in]
          n344 = To Single Precision Float(number=w498) -> (single precision float=w496:sgl[])
          n345 = call "Vp-1D-temp.vi"("array in"=w496, "command"=enum16{"get", "set", "clear", "append"}."set") -> ()  [unwired: 2 in, 2 out]
        }
        frame 43 {
          n346 = Index Array(array=w508, index (row)=2) -> (element=w520:i16[])  [unwired: 1 in]
          n347 = Index Array(array=w508, index (row)=0) -> (element=w522:i16[])  [unwired: 1 in]
          n348 = Index Array(array=w508, index (row)=1) -> (element=w521:i16[])  [unwired: 1 in]
          n349 = To Single Precision Float(number=w522) -> (single precision float=w517:sgl[])
          n350 = To Single Precision Float(number=w520) -> (single precision float=w514:sgl[])
          n351 = To Single Precision Float(number=w521) -> (single precision float=w515:sgl[])
          n352 = call "CH1-1D-temp.vi"("array in"=w517, "command"=enum16{"get", "set", "clear", "append"}."set") -> ()  [unwired: 2 in, 2 out]
          n353 = call "CH2-1D-temp.vi"("array in"=w515, "command"=enum16{"get", "set", "clear", "append"}."set") -> ()  [unwired: 2 in, 2 out]
          n354 = call "Y-1D-temp.vi"("array in"=w514, "command"=enum16{"get", "set", "clear", "append"}."set") -> ()  [unwired: 2 in, 2 out]
          n355 = Index Array(array=w508, index (row)=4) -> (element=w511:i16[])  [unwired: 1 in]
          n356 = To Single Precision Float(number=w511) -> (single precision float=w509:sgl[])
          n357 = call "Vp-1D-temp.vi"("array in"=w509, "command"=enum16{"get", "set", "clear", "append"}."set") -> ()  [unwired: 2 in, 2 out]
        }
        frame 44 {
          n358 = Index Array(array=w525, index (row)=1) -> (element=w535:i16[])  [unwired: 1 in]
          n359 = Index Array(array=w525, index (row)=0) -> (element=w536:i16[])  [unwired: 1 in]
          n360 = To Single Precision Float(number=w535) -> (single precision float=w530:sgl[])
          n361 = To Single Precision Float(number=w536) -> (single precision float=w532:sgl[])
          n362 = call "Y-1D-temp.vi"("array in"=w530, "command"=enum16{"get", "set", "clear", "append"}."set") -> ()  [unwired: 2 in, 2 out]
          n363 = Index Array(array=w525, index (row)=3) -> (element=w528:i16[])  [unwired: 1 in]
          n364 = call "X-1D-temp.vi"("array in"=w532, "command"=enum16{"get", "set", "clear", "append"}."set") -> ()  [unwired: 2 in, 2 out]
          n365 = To Single Precision Float(number=w528) -> (single precision float=w526:sgl[])
          n366 = call "Vp-1D-temp.vi"("array in"=w526, "command"=enum16{"get", "set", "clear", "append"}."set") -> ()  [unwired: 2 in, 2 out]
        }
        frame 45 {
          n367 = Index Array(array=w538, index (row)=0) -> (element=w552:i16[])  [unwired: 1 in]
          n368 = Index Array(array=w538, index (row)=1) -> (element=w551:i16[])  [unwired: 1 in]
          n369 = Index Array(array=w538, index (row)=2) -> (element=w550:i16[])  [unwired: 1 in]
          n370 = To Single Precision Float(number=w552) -> (single precision float=w547:sgl[])
          n371 = To Single Precision Float(number=w551) -> (single precision float=w545:sgl[])
          n372 = To Single Precision Float(number=w550) -> (single precision float=w543:sgl[])
          n373 = Index Array(array=w538, index (row)=4) -> (element=w541:i16[])  [unwired: 1 in]
          n374 = call "CH1-1D-temp.vi"("array in"=w547, "command"=enum16{"get", "set", "clear", "append"}."set") -> ()  [unwired: 2 in, 2 out]
          n375 = call "X-1D-temp.vi"("array in"=w545, "command"=enum16{"get", "set", "clear", "append"}."set") -> ()  [unwired: 2 in, 2 out]
          n376 = call "Y-1D-temp.vi"("array in"=w543, "command"=enum16{"get", "set", "clear", "append"}."set") -> ()  [unwired: 2 in, 2 out]
          n377 = To Single Precision Float(number=w541) -> (single precision float=w539:sgl[])
          n378 = call "Vp-1D-temp.vi"("array in"=w539, "command"=enum16{"get", "set", "clear", "append"}."set") -> ()  [unwired: 2 in, 2 out]
        }
        frame 46 {
          n379 = Index Array(array=w555, index (row)=0) -> (element=w569:i16[])  [unwired: 1 in]
          n380 = Index Array(array=w555, index (row)=1) -> (element=w568:i16[])  [unwired: 1 in]
          n381 = Index Array(array=w555, index (row)=4) -> (element=w558:i16[])  [unwired: 1 in]
          n382 = Index Array(array=w555, index (row)=2) -> (element=w567:i16[])  [unwired: 1 in]
          n383 = To Single Precision Float(number=w569) -> (single precision float=w564:sgl[])
          n384 = To Single Precision Float(number=w558) -> (single precision float=w556:sgl[])
          n385 = To Single Precision Float(number=w568) -> (single precision float=w562:sgl[])
          n386 = To Single Precision Float(number=w567) -> (single precision float=w560:sgl[])
          n387 = call "CH2-1D-temp.vi"("array in"=w564, "command"=enum16{"get", "set", "clear", "append"}."set") -> ()  [unwired: 2 in, 2 out]
          n388 = call "Vp-1D-temp.vi"("array in"=w556, "command"=enum16{"get", "set", "clear", "append"}."set") -> ()  [unwired: 2 in, 2 out]
          n389 = call "X-1D-temp.vi"("array in"=w562, "command"=enum16{"get", "set", "clear", "append"}."set") -> ()  [unwired: 2 in, 2 out]
          n390 = call "Y-1D-temp.vi"("array in"=w560, "command"=enum16{"get", "set", "clear", "append"}."set") -> ()  [unwired: 2 in, 2 out]
        }
        frame 47 {
          n391 = Index Array(array=w572, index (row)=0) -> (element=w589:i16[])  [unwired: 1 in]
          n392 = Index Array(array=w572, index (row)=1) -> (element=w588:i16[])  [unwired: 1 in]
          n393 = Index Array(array=w572, index (row)=2) -> (element=w587:i16[])  [unwired: 1 in]
          n394 = Index Array(array=w572, index (row)=3) -> (element=w586:i16[])  [unwired: 1 in]
          n395 = Index Array(array=w572, index (row)=5) -> (element=w575:i16[])  [unwired: 1 in]
          n396 = To Single Precision Float(number=w589) -> (single precision float=w583:sgl[])
          n397 = To Single Precision Float(number=w588) -> (single precision float=w581:sgl[])
          n398 = To Single Precision Float(number=w587) -> (single precision float=w579:sgl[])
          n399 = To Single Precision Float(number=w586) -> (single precision float=w577:sgl[])
          n400 = To Single Precision Float(number=w575) -> (single precision float=w573:sgl[])
          n401 = call "Vp-1D-temp.vi"("array in"=w573, "command"=enum16{"get", "set", "clear", "append"}."set") -> ()  [unwired: 2 in, 2 out]
          n402 = call "X-1D-temp.vi"("array in"=w579, "command"=enum16{"get", "set", "clear", "append"}."set") -> ()  [unwired: 2 in, 2 out]
          n403 = call "Y-1D-temp.vi"("array in"=w577, "command"=enum16{"get", "set", "clear", "append"}."set") -> ()  [unwired: 2 in, 2 out]
          n404 = call "CH1-1D-temp.vi"("array in"=w583, "command"=enum16{"get", "set", "clear", "append"}."set") -> ()  [unwired: 2 in, 2 out]
          n405 = call "CH2-1D-temp.vi"("array in"=w581, "command"=enum16{"get", "set", "clear", "append"}."set") -> ()  [unwired: 2 in, 2 out]
        }
        frame 48 {
          n406 = Index Array(array=w593, index (row)=0) -> (element=w599:i16[])  [unwired: 1 in]
          n407 = Index Array(array=w593, index (row)=1) -> (element=w598:i16[])  [unwired: 1 in]
          n408 = To Single Precision Float(number=w599) -> (single precision float=w596:sgl[])
          n409 = To Single Precision Float(number=w598) -> (single precision float=w594:sgl[])
          n410 = call "Ip-1D-temp.vi"("array in"=w596, "command"=enum16{"get", "set", "clear", "append"}."set") -> ()  [unwired: 2 in, 2 out]
          n411 = call "Vp-1D-temp.vi"("array in"=w594, "command"=enum16{"get", "set", "clear", "append"}."set") -> ()  [unwired: 2 in, 2 out]
        }
        frame 49 {
          n412 = Index Array(array=w602, index (row)=0) -> (element=w613:i16[])  [unwired: 1 in]
          n413 = To Single Precision Float(number=w613) -> (single precision float=w611:sgl[])
          n414 = call "CH1-1D-temp.vi"("array in"=w611, "command"=enum16{"get", "set", "clear", "append"}."set") -> ()  [unwired: 2 in, 2 out]
          n415 = Index Array(array=w602, index (row)=1) -> (element=w608:i16[])  [unwired: 1 in]
          n416 = Index Array(array=w602, index (row)=2) -> (element=w607:i16[])  [unwired: 1 in]
          n417 = To Single Precision Float(number=w608) -> (single precision float=w605:sgl[])
          n418 = To Single Precision Float(number=w607) -> (single precision float=w603:sgl[])
          n419 = call "Ip-1D-temp.vi"("array in"=w605, "command"=enum16{"get", "set", "clear", "append"}."set") -> ()  [unwired: 2 in, 2 out]
          n420 = call "Vp-1D-temp.vi"("array in"=w603, "command"=enum16{"get", "set", "clear", "append"}."set") -> ()  [unwired: 2 in, 2 out]
        }
        frame 50 {
          n421 = Index Array(array=w615, index (row)=0) -> (element=w626:i16[])  [unwired: 1 in]
          n422 = To Single Precision Float(number=w626) -> (single precision float=w625:sgl[])
          n423 = Index Array(array=w615, index (row)=1) -> (element=w621:i16[])  [unwired: 1 in]
          n424 = Index Array(array=w615, index (row)=2) -> (element=w620:i16[])  [unwired: 1 in]
          n425 = call "CH2-1D-temp.vi"("array in"=w625, "command"=enum16{"get", "set", "clear", "append"}."set") -> ()  [unwired: 2 in, 2 out]
          n426 = To Single Precision Float(number=w621) -> (single precision float=w618:sgl[])
          n427 = To Single Precision Float(number=w620) -> (single precision float=w616:sgl[])
          n428 = call "Ip-1D-temp.vi"("array in"=w618, "command"=enum16{"get", "set", "clear", "append"}."set") -> ()  [unwired: 2 in, 2 out]
          n429 = call "Vp-1D-temp.vi"("array in"=w616, "command"=enum16{"get", "set", "clear", "append"}."set") -> ()  [unwired: 2 in, 2 out]
        }
        frame 51 {
          n430 = Index Array(array=w628, index (row)=0) -> (element=w642:i16[])  [unwired: 1 in]
          n431 = Index Array(array=w628, index (row)=1) -> (element=w641:i16[])  [unwired: 1 in]
          n432 = To Single Precision Float(number=w642) -> (single precision float=w639:sgl[])
          n433 = To Single Precision Float(number=w641) -> (single precision float=w637:sgl[])
          n434 = call "CH1-1D-temp.vi"("array in"=w639, "command"=enum16{"get", "set", "clear", "append"}."set") -> ()  [unwired: 2 in, 2 out]
          n435 = call "CH2-1D-temp.vi"("array in"=w637, "command"=enum16{"get", "set", "clear", "append"}."set") -> ()  [unwired: 2 in, 2 out]
          n436 = Index Array(array=w628, index (row)=2) -> (element=w634:i16[])  [unwired: 1 in]
          n437 = Index Array(array=w628, index (row)=3) -> (element=w633:i16[])  [unwired: 1 in]
          n438 = To Single Precision Float(number=w634) -> (single precision float=w631:sgl[])
          n439 = To Single Precision Float(number=w633) -> (single precision float=w629:sgl[])
          n440 = call "Ip-1D-temp.vi"("array in"=w631, "command"=enum16{"get", "set", "clear", "append"}."set") -> ()  [unwired: 2 in, 2 out]
          n441 = call "Vp-1D-temp.vi"("array in"=w629, "command"=enum16{"get", "set", "clear", "append"}."set") -> ()  [unwired: 2 in, 2 out]
        }
        frame 52 {
          n442 = Index Array(array=w645, index (row)=0) -> (element=w656:i16[])  [unwired: 1 in]
          n443 = To Single Precision Float(number=w656) -> (single precision float=w654:sgl[])
          n444 = Index Array(array=w645, index (row)=1) -> (element=w651:i16[])  [unwired: 1 in]
          n445 = Index Array(array=w645, index (row)=2) -> (element=w650:i16[])  [unwired: 1 in]
          n446 = call "X-1D-temp.vi"("array in"=w654, "command"=enum16{"get", "set", "clear", "append"}."set") -> ()  [unwired: 2 in, 2 out]
          n447 = To Single Precision Float(number=w651) -> (single precision float=w648:sgl[])
          n448 = To Single Precision Float(number=w650) -> (single precision float=w646:sgl[])
          n449 = call "Ip-1D-temp.vi"("array in"=w648, "command"=enum16{"get", "set", "clear", "append"}."set") -> ()  [unwired: 2 in, 2 out]
          n450 = call "Vp-1D-temp.vi"("array in"=w646, "command"=enum16{"get", "set", "clear", "append"}."set") -> ()  [unwired: 2 in, 2 out]
        }
        frame 53 {
          n451 = Index Array(array=w658, index (row)=0) -> (element=w672:i16[])  [unwired: 1 in]
          n452 = Index Array(array=w658, index (row)=1) -> (element=w671:i16[])  [unwired: 1 in]
          n453 = To Single Precision Float(number=w672) -> (single precision float=w669:sgl[])
          n454 = To Single Precision Float(number=w671) -> (single precision float=w667:sgl[])
          n455 = Index Array(array=w658, index (row)=2) -> (element=w664:i16[])  [unwired: 1 in]
          n456 = Index Array(array=w658, index (row)=3) -> (element=w663:i16[])  [unwired: 1 in]
          n457 = call "X-1D-temp.vi"("array in"=w667, "command"=enum16{"get", "set", "clear", "append"}."set") -> ()  [unwired: 2 in, 2 out]
          n458 = call "CH1-1D-temp.vi"("array in"=w669, "command"=enum16{"get", "set", "clear", "append"}."set") -> ()  [unwired: 2 in, 2 out]
          n459 = To Single Precision Float(number=w664) -> (single precision float=w661:sgl[])
          n460 = To Single Precision Float(number=w663) -> (single precision float=w659:sgl[])
          n461 = call "Ip-1D-temp.vi"("array in"=w661, "command"=enum16{"get", "set", "clear", "append"}."set") -> ()  [unwired: 2 in, 2 out]
          n462 = call "Vp-1D-temp.vi"("array in"=w659, "command"=enum16{"get", "set", "clear", "append"}."set") -> ()  [unwired: 2 in, 2 out]
        }
        frame 54 {
          n463 = Index Array(array=w675, index (row)=0) -> (element=w689:i16[])  [unwired: 1 in]
          n464 = Index Array(array=w675, index (row)=1) -> (element=w688:i16[])  [unwired: 1 in]
          n465 = To Single Precision Float(number=w689) -> (single precision float=w686:sgl[])
          n466 = To Single Precision Float(number=w688) -> (single precision float=w684:sgl[])
          n467 = Index Array(array=w675, index (row)=2) -> (element=w681:i16[])  [unwired: 1 in]
          n468 = Index Array(array=w675, index (row)=3) -> (element=w680:i16[])  [unwired: 1 in]
          n469 = call "CH2-1D-temp.vi"("array in"=w686, "command"=enum16{"get", "set", "clear", "append"}."set") -> ()  [unwired: 2 in, 2 out]
          n470 = To Single Precision Float(number=w681) -> (single precision float=w678:sgl[])
          n471 = call "X-1D-temp.vi"("array in"=w684, "command"=enum16{"get", "set", "clear", "append"}."set") -> ()  [unwired: 2 in, 2 out]
          n472 = To Single Precision Float(number=w680) -> (single precision float=w676:sgl[])
          n473 = call "Ip-1D-temp.vi"("array in"=w678, "command"=enum16{"get", "set", "clear", "append"}."set") -> ()  [unwired: 2 in, 2 out]
          n474 = call "Vp-1D-temp.vi"("array in"=w676, "command"=enum16{"get", "set", "clear", "append"}."set") -> ()  [unwired: 2 in, 2 out]
        }
        frame 55 {
          n475 = Index Array(array=w692, index (row)=0) -> (element=w709:i16[])  [unwired: 1 in]
          n476 = Index Array(array=w692, index (row)=1) -> (element=w708:i16[])  [unwired: 1 in]
          n477 = Index Array(array=w692, index (row)=2) -> (element=w707:i16[])  [unwired: 1 in]
          n478 = To Single Precision Float(number=w709) -> (single precision float=w705:sgl[])
          n479 = To Single Precision Float(number=w708) -> (single precision float=w703:sgl[])
          n480 = To Single Precision Float(number=w707) -> (single precision float=w701:sgl[])
          n481 = call "CH1-1D-temp.vi"("array in"=w705, "command"=enum16{"get", "set", "clear", "append"}."set") -> ()  [unwired: 2 in, 2 out]
          n482 = Index Array(array=w692, index (row)=3) -> (element=w698:i16[])  [unwired: 1 in]
          n483 = call "CH2-1D-temp.vi"("array in"=w703, "command"=enum16{"get", "set", "clear", "append"}."set") -> ()  [unwired: 2 in, 2 out]
          n484 = Index Array(array=w692, index (row)=4) -> (element=w697:i16[])  [unwired: 1 in]
          n485 = call "X-1D-temp.vi"("array in"=w701, "command"=enum16{"get", "set", "clear", "append"}."set") -> ()  [unwired: 2 in, 2 out]
          n486 = To Single Precision Float(number=w698) -> (single precision float=w695:sgl[])
          n487 = To Single Precision Float(number=w697) -> (single precision float=w693:sgl[])
          n488 = call "Ip-1D-temp.vi"("array in"=w695, "command"=enum16{"get", "set", "clear", "append"}."set") -> ()  [unwired: 2 in, 2 out]
          n489 = call "Vp-1D-temp.vi"("array in"=w693, "command"=enum16{"get", "set", "clear", "append"}."set") -> ()  [unwired: 2 in, 2 out]
        }
        frame 56 {
          n490 = Index Array(array=w713, index (row)=0) -> (element=w725:i16[])  [unwired: 1 in]
          n491 = To Single Precision Float(number=w725) -> (single precision float=w722:sgl[])
          n492 = call "Y-1D-temp.vi"("array in"=w722, "command"=enum16{"get", "set", "clear", "append"}."set") -> ()  [unwired: 2 in, 2 out]
          n493 = Index Array(array=w713, index (row)=1) -> (element=w719:i16[])  [unwired: 1 in]
          n494 = Index Array(array=w713, index (row)=2) -> (element=w718:i16[])  [unwired: 1 in]
          n495 = To Single Precision Float(number=w719) -> (single precision float=w716:sgl[])
          n496 = To Single Precision Float(number=w718) -> (single precision float=w714:sgl[])
          n497 = call "Ip-1D-temp.vi"("array in"=w716, "command"=enum16{"get", "set", "clear", "append"}."set") -> ()  [unwired: 2 in, 2 out]
          n498 = call "Vp-1D-temp.vi"("array in"=w714, "command"=enum16{"get", "set", "clear", "append"}."set") -> ()  [unwired: 2 in, 2 out]
        }
        frame 57 {
          n499 = Index Array(array=w726, index (row)=1) -> (element=w740:i16[])  [unwired: 1 in]
          n500 = Index Array(array=w726, index (row)=0) -> (element=w741:i16[])  [unwired: 1 in]
          n501 = To Single Precision Float(number=w740) -> (single precision float=w735:sgl[])
          n502 = To Single Precision Float(number=w741) -> (single precision float=w737:sgl[])
          n503 = call "Y-1D-temp.vi"("array in"=w735, "command"=enum16{"get", "set", "clear", "append"}."set") -> ()  [unwired: 2 in, 2 out]
          n504 = call "CH1-1D-temp.vi"("array in"=w737, "command"=enum16{"get", "set", "clear", "append"}."set") -> ()  [unwired: 2 in, 2 out]
          n505 = Index Array(array=w726, index (row)=2) -> (element=w732:i16[])  [unwired: 1 in]
          n506 = Index Array(array=w726, index (row)=3) -> (element=w731:i16[])  [unwired: 1 in]
          n507 = To Single Precision Float(number=w732) -> (single precision float=w729:sgl[])
          n508 = To Single Precision Float(number=w731) -> (single precision float=w727:sgl[])
          n509 = call "Ip-1D-temp.vi"("array in"=w729, "command"=enum16{"get", "set", "clear", "append"}."set") -> ()  [unwired: 2 in, 2 out]
          n510 = call "Vp-1D-temp.vi"("array in"=w727, "command"=enum16{"get", "set", "clear", "append"}."set") -> ()  [unwired: 2 in, 2 out]
        }
        frame 58 {
          n511 = Index Array(array=w743, index (row)=1) -> (element=w757:i16[])  [unwired: 1 in]
          n512 = Index Array(array=w743, index (row)=0) -> (element=w758:i16[])  [unwired: 1 in]
          n513 = To Single Precision Float(number=w757) -> (single precision float=w752:sgl[])
          n514 = To Single Precision Float(number=w758) -> (single precision float=w755:sgl[])
          n515 = call "Y-1D-temp.vi"("array in"=w752, "command"=enum16{"get", "set", "clear", "append"}."set") -> ()  [unwired: 2 in, 2 out]
          n516 = call "CH2-1D-temp.vi"("array in"=w755, "command"=enum16{"get", "set", "clear", "append"}."set") -> ()  [unwired: 2 in, 2 out]
          n517 = Index Array(array=w743, index (row)=2) -> (element=w749:i16[])  [unwired: 1 in]
          n518 = Index Array(array=w743, index (row)=3) -> (element=w748:i16[])  [unwired: 1 in]
          n519 = To Single Precision Float(number=w749) -> (single precision float=w746:sgl[])
          n520 = To Single Precision Float(number=w748) -> (single precision float=w744:sgl[])
          n521 = call "Ip-1D-temp.vi"("array in"=w746, "command"=enum16{"get", "set", "clear", "append"}."set") -> ()  [unwired: 2 in, 2 out]
          n522 = call "Vp-1D-temp.vi"("array in"=w744, "command"=enum16{"get", "set", "clear", "append"}."set") -> ()  [unwired: 2 in, 2 out]
        }
        frame 59 {
          n523 = Index Array(array=w760, index (row)=2) -> (element=w776:i16[])  [unwired: 1 in]
          n524 = Index Array(array=w760, index (row)=0) -> (element=w778:i16[])  [unwired: 1 in]
          n525 = Index Array(array=w760, index (row)=1) -> (element=w777:i16[])  [unwired: 1 in]
          n526 = To Single Precision Float(number=w778) -> (single precision float=w773:sgl[])
          n527 = To Single Precision Float(number=w776) -> (single precision float=w770:sgl[])
          n528 = To Single Precision Float(number=w777) -> (single precision float=w771:sgl[])
          n529 = call "CH1-1D-temp.vi"("array in"=w773, "command"=enum16{"get", "set", "clear", "append"}."set") -> ()  [unwired: 2 in, 2 out]
          n530 = call "CH2-1D-temp.vi"("array in"=w771, "command"=enum16{"get", "set", "clear", "append"}."set") -> ()  [unwired: 2 in, 2 out]
          n531 = Index Array(array=w760, index (row)=3) -> (element=w766:i16[])  [unwired: 1 in]
          n532 = call "Y-1D-temp.vi"("array in"=w770, "command"=enum16{"get", "set", "clear", "append"}."set") -> ()  [unwired: 2 in, 2 out]
          n533 = Index Array(array=w760, index (row)=4) -> (element=w765:i16[])  [unwired: 1 in]
          n534 = To Single Precision Float(number=w766) -> (single precision float=w763:sgl[])
          n535 = To Single Precision Float(number=w765) -> (single precision float=w761:sgl[])
          n536 = call "Ip-1D-temp.vi"("array in"=w763, "command"=enum16{"get", "set", "clear", "append"}."set") -> ()  [unwired: 2 in, 2 out]
          n537 = call "Vp-1D-temp.vi"("array in"=w761, "command"=enum16{"get", "set", "clear", "append"}."set") -> ()  [unwired: 2 in, 2 out]
        }
        frame 60 {
          n538 = Index Array(array=w781, index (row)=1) -> (element=w795:i16[])  [unwired: 1 in]
          n539 = Index Array(array=w781, index (row)=0) -> (element=w796:i16[])  [unwired: 1 in]
          n540 = To Single Precision Float(number=w795) -> (single precision float=w790:sgl[])
          n541 = To Single Precision Float(number=w796) -> (single precision float=w792:sgl[])
          n542 = call "Y-1D-temp.vi"("array in"=w790, "command"=enum16{"get", "set", "clear", "append"}."set") -> ()  [unwired: 2 in, 2 out]
          n543 = Index Array(array=w781, index (row)=2) -> (element=w787:i16[])  [unwired: 1 in]
          n544 = Index Array(array=w781, index (row)=3) -> (element=w786:i16[])  [unwired: 1 in]
          n545 = call "X-1D-temp.vi"("array in"=w792, "command"=enum16{"get", "set", "clear", "append"}."set") -> ()  [unwired: 2 in, 2 out]
          n546 = To Single Precision Float(number=w787) -> (single precision float=w784:sgl[])
          n547 = To Single Precision Float(number=w786) -> (single precision float=w782:sgl[])
          n548 = call "Ip-1D-temp.vi"("array in"=w784, "command"=enum16{"get", "set", "clear", "append"}."set") -> ()  [unwired: 2 in, 2 out]
          n549 = call "Vp-1D-temp.vi"("array in"=w782, "command"=enum16{"get", "set", "clear", "append"}."set") -> ()  [unwired: 2 in, 2 out]
        }
        frame 61 {
          n550 = Index Array(array=w798, index (row)=0) -> (element=w816:i16[])  [unwired: 1 in]
          n551 = Index Array(array=w798, index (row)=1) -> (element=w815:i16[])  [unwired: 1 in]
          n552 = Index Array(array=w798, index (row)=2) -> (element=w814:i16[])  [unwired: 1 in]
          n553 = To Single Precision Float(number=w816) -> (single precision float=w811:sgl[])
          n554 = To Single Precision Float(number=w815) -> (single precision float=w809:sgl[])
          n555 = To Single Precision Float(number=w814) -> (single precision float=w807:sgl[])
          n556 = Index Array(array=w798, index (row)=3) -> (element=w804:i16[])  [unwired: 1 in]
          n557 = Index Array(array=w798, index (row)=4) -> (element=w803:i16[])  [unwired: 1 in]
          n558 = call "CH1-1D-temp.vi"("array in"=w811, "command"=enum16{"get", "set", "clear", "append"}."set") -> ()  [unwired: 2 in, 2 out]
          n559 = call "X-1D-temp.vi"("array in"=w809, "command"=enum16{"get", "set", "clear", "append"}."set") -> ()  [unwired: 2 in, 2 out]
          n560 = call "Y-1D-temp.vi"("array in"=w807, "command"=enum16{"get", "set", "clear", "append"}."set") -> ()  [unwired: 2 in, 2 out]
          n561 = To Single Precision Float(number=w804) -> (single precision float=w801:sgl[])
          n562 = To Single Precision Float(number=w803) -> (single precision float=w799:sgl[])
          n563 = call "Ip-1D-temp.vi"("array in"=w801, "command"=enum16{"get", "set", "clear", "append"}."set") -> ()  [unwired: 2 in, 2 out]
          n564 = call "Vp-1D-temp.vi"("array in"=w799, "command"=enum16{"get", "set", "clear", "append"}."set") -> ()  [unwired: 2 in, 2 out]
        }
        frame 62 {
          n565 = Index Array(array=w819, index (row)=3) -> (element=w825:i16[])  [unwired: 1 in]
          n566 = Index Array(array=w819, index (row)=0) -> (element=w837:i16[])  [unwired: 1 in]
          n567 = Index Array(array=w819, index (row)=1) -> (element=w836:i16[])  [unwired: 1 in]
          n568 = Index Array(array=w819, index (row)=4) -> (element=w824:i16[])  [unwired: 1 in]
          n569 = Index Array(array=w819, index (row)=2) -> (element=w835:i16[])  [unwired: 1 in]
          n570 = To Single Precision Float(number=w825) -> (single precision float=w822:sgl[])
          n571 = To Single Precision Float(number=w837) -> (single precision float=w832:sgl[])
          n572 = To Single Precision Float(number=w824) -> (single precision float=w820:sgl[])
          n573 = To Single Precision Float(number=w836) -> (single precision float=w830:sgl[])
          n574 = To Single Precision Float(number=w835) -> (single precision float=w828:sgl[])
          n575 = call "CH2-1D-temp.vi"("array in"=w832, "command"=enum16{"get", "set", "clear", "append"}."set") -> ()  [unwired: 2 in, 2 out]
          n576 = call "Ip-1D-temp.vi"("array in"=w822, "command"=enum16{"get", "set", "clear", "append"}."set") -> ()  [unwired: 2 in, 2 out]
          n577 = call "Vp-1D-temp.vi"("array in"=w820, "command"=enum16{"get", "set", "clear", "append"}."set") -> ()  [unwired: 2 in, 2 out]
          n578 = call "X-1D-temp.vi"("array in"=w830, "command"=enum16{"get", "set", "clear", "append"}."set") -> ()  [unwired: 2 in, 2 out]
          n579 = call "Y-1D-temp.vi"("array in"=w828, "command"=enum16{"get", "set", "clear", "append"}."set") -> ()  [unwired: 2 in, 2 out]
        }
        frame 63 {
          n580 = Index Array(array=w840, index (row)=0) -> (element=w861:i16[])  [unwired: 1 in]
          n581 = Index Array(array=w840, index (row)=1) -> (element=w860:i16[])  [unwired: 1 in]
          n582 = Index Array(array=w840, index (row)=2) -> (element=w859:i16[])  [unwired: 1 in]
          n583 = Index Array(array=w840, index (row)=3) -> (element=w858:i16[])  [unwired: 1 in]
          n584 = Index Array(array=w840, index (row)=4) -> (element=w846:i16[])  [unwired: 1 in]
          n585 = Index Array(array=w840, index (row)=5) -> (element=w845:i16[])  [unwired: 1 in]
          n586 = To Single Precision Float(number=w861) -> (single precision float=w855:sgl[])
          n587 = To Single Precision Float(number=w860) -> (single precision float=w853:sgl[])
          n588 = To Single Precision Float(number=w846) -> (single precision float=w843:sgl[])
          n589 = To Single Precision Float(number=w859) -> (single precision float=w851:sgl[])
          n590 = To Single Precision Float(number=w858) -> (single precision float=w849:sgl[])
          n591 = To Single Precision Float(number=w845) -> (single precision float=w841:sgl[])
          n592 = call "Ip-1D-temp.vi"("array in"=w843, "command"=enum16{"get", "set", "clear", "append"}."set") -> ()  [unwired: 2 in, 2 out]
          n593 = call "Vp-1D-temp.vi"("array in"=w841, "command"=enum16{"get", "set", "clear", "append"}."set") -> ()  [unwired: 2 in, 2 out]
          n594 = call "X-1D-temp.vi"("array in"=w851, "command"=enum16{"get", "set", "clear", "append"}."set") -> ()  [unwired: 2 in, 2 out]
          n595 = call "Y-1D-temp.vi"("array in"=w849, "command"=enum16{"get", "set", "clear", "append"}."set") -> ()  [unwired: 2 in, 2 out]
          n596 = call "CH1-1D-temp.vi"("array in"=w855, "command"=enum16{"get", "set", "clear", "append"}."set") -> ()  [unwired: 2 in, 2 out]
          n597 = call "CH2-1D-temp.vi"("array in"=w853, "command"=enum16{"get", "set", "clear", "append"}."set") -> ()  [unwired: 2 in, 2 out]
        }
      }
    }
  }
